vi "GenerateFrictionModel.vi"() -> (0 "Friction Model Parameters":T1(array[cluster]))   [LabVIEW 2013]
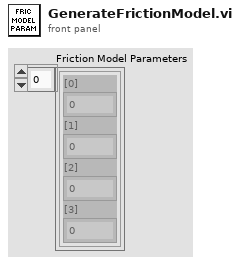
[diagram p1: front panel]
types:
  T1 = cluster{"[0]":dbl, "[1]":dbl, "[2]":dbl, "[3]":dbl}[]
  T2 = cluster{"[0]":dbl, "[1]":dbl, "[2]":dbl, "[3]":dbl}
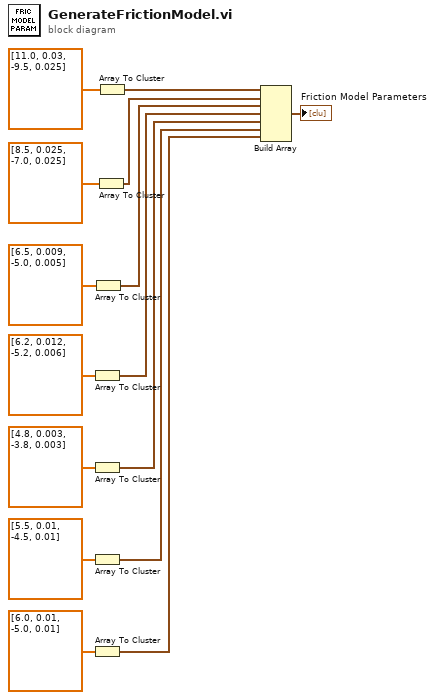
[diagram p0: block diagram]
diagram:
  n1 = Array To Cluster(array=dbl[] [6.2, 0.012, -5.2, 0.006]) -> (cluster=w5:T2)
  n2 = Array To Cluster(array=dbl[] [4.8, 0.003, -3.8, 0.003]) -> (cluster=w4:T2)
  n3 = Array To Cluster(array=dbl[] [5.5, 0.01, -4.5, 0.01]) -> (cluster=w3:T2)
  n4 = Array To Cluster(array=dbl[] [6.0, 0.01, -5.0, 0.01]) -> (cluster=w2:T2)
  n5 = Array To Cluster(array=dbl[] [6.5, 0.009, -5.0, 0.005]) -> (cluster=w10:T2)
  n6 = Array To Cluster(array=dbl[] [8.5, 0.025, -7.0, 0.025]) -> (cluster=w12:T2)
  n7 = Array To Cluster(array=dbl[] [11.0, 0.03, -9.5, 0.025]) -> (cluster=w14:T2)
  n8 = Build Array(w14, w12, w10, w5, w4, w3, w2) -> (→"Friction Model Parameters":T1)
